vi "Sine.vi"() -> ()   [LabVIEW 2024]
uses:
  <vilib>/Analysis/1siggen.llb/Ramp Pattern by Samples.vi
  <vilib>/measure/NI_MABase.lvlib
  <vilib>/Analysis/NI_AALBase.lvlib
panel:
  out "Sine Graph":waveform(dbl)(graph)
  in  "Stop Button":bool
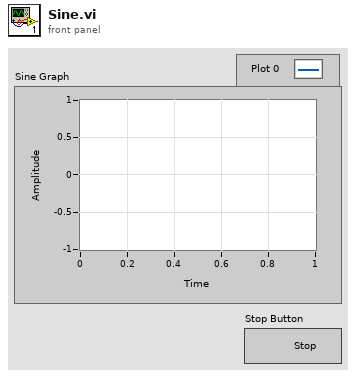
[diagram p1: front panel]
types:
  T1 = enum16{"Sine Wave", "Triangle Wave", "Square Wave", "Sawtooth Wave"}
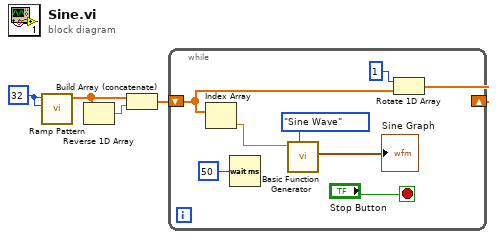
[diagram p0: block diagram]
diagram:
  w2 = 32 ("samples")
  n1 = call-poly <vilib>:"Ramp Pattern.vi"("end"=w2, "samples"=w2) -> ("Ramp Pattern"=w1:dbl[])  [unwired: 8 in, 1 out]
  n2 = Reverse 1D Array(array=w1) -> (reversed array=w4:dbl[])
  n3 = Build Array (concatenate)(w1, w4) -> (w3:dbl[])
  n4 = while {
    shift-right: [w8] -> _
    shift-left: w3 -> [w5]
    stop <- "Stop Button" stop-if-true
    n5 = Index Array(array=w5) -> (element=w7:dbl)  [unwired: 1 in]
    n6 = Wait (ms)(milliseconds to wait=u32 50) -> ()  [unwired: 1 out]
    n7 = call <vilib>:"Basic Function Generator.vi"("signal type"=T1."Sine Wave", "frequency"=w7) -> ("signal out"=→"Sine Graph":waveform(dbl))  [unwired: 7 in, 2 out]
    n8 = Rotate 1D Array(1:w5, 2:1 ("n")) -> (0:w8:dbl[])
  }
